vi "S8300E_BP_VLAN_WIH.vi"() -> ()   [LabVIEW 2011]
panel:
  out "PreLog1":string
  out "prelog2":string
  out "log2":string
  out "FinalLog1":string
  out "LOG1":string
  out "Finallog2":string
  out "Test CMD":T1(array[cluster])
  out "Init CMD":T2(array[cluster])
  out "VISA Handle Array":refnum<visa-resource-name>[](array[refnum])
  out "VISA6":refnum<visa-resource-name>
  out "VISA9":refnum<visa-resource-name>
  out "BEGIN TIME":u32
  out "進行狀況":string
  # "Error Code:BP-VLAN"
  # "S8300E BackPlane  VLAN"
  # "2015-5-28"
  # "PC Com9 Baud  115200 -->S8300E MB\nPC COM6 Baud 115200 -->Test Board UART"
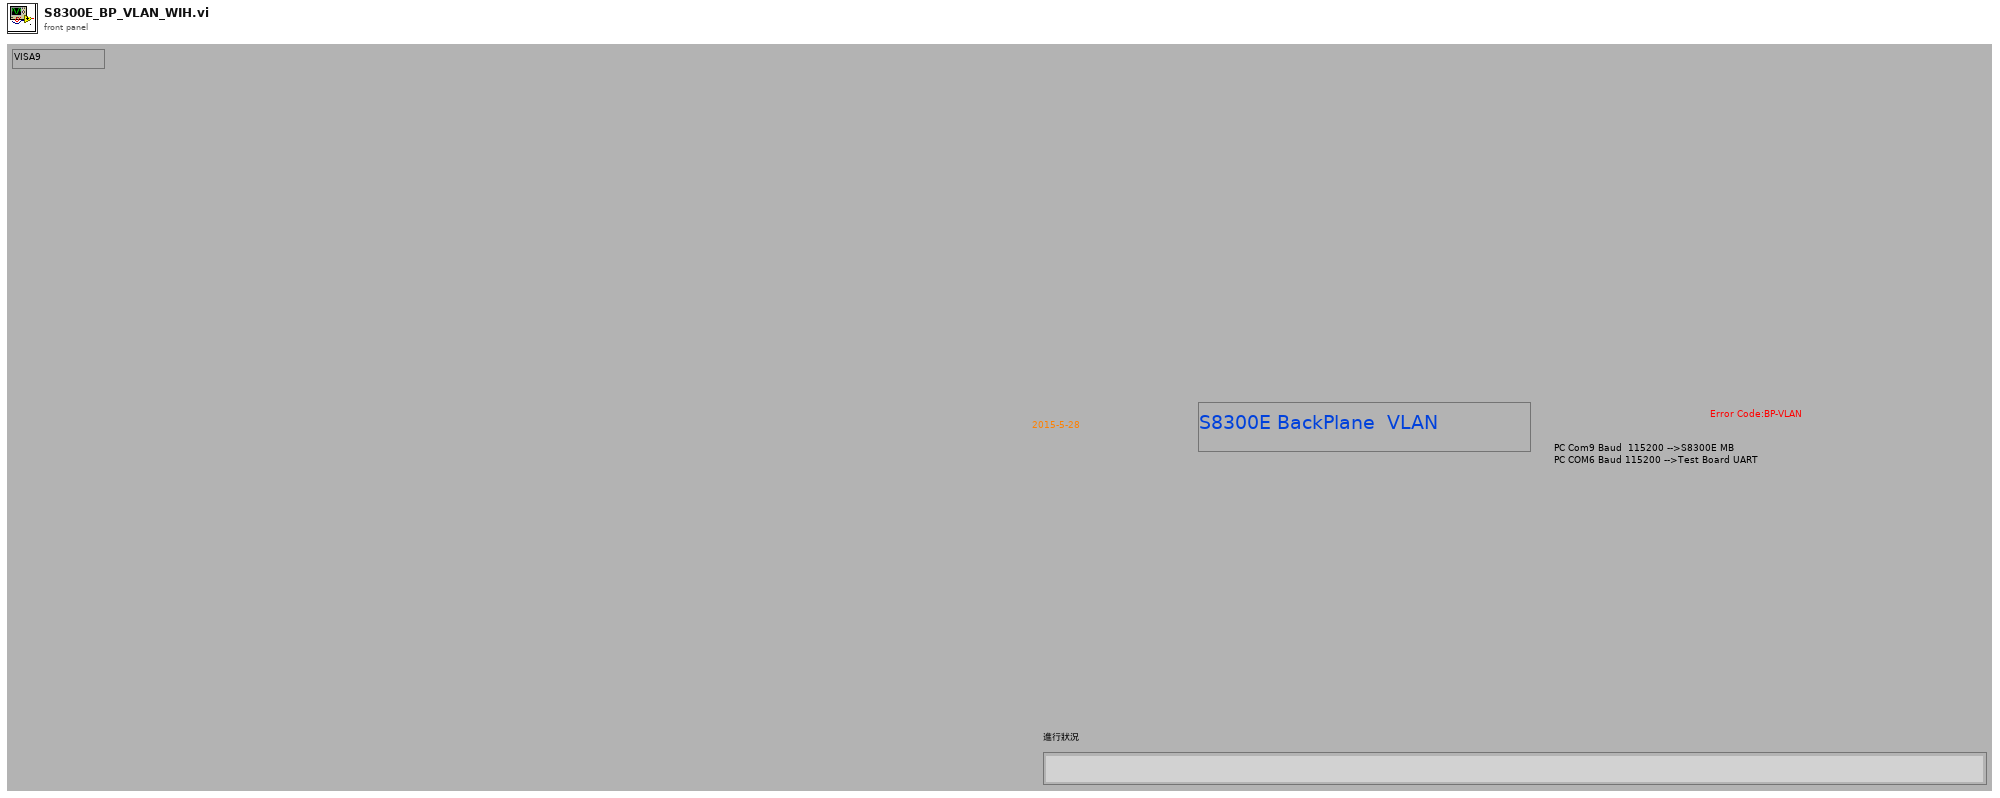
[diagram p1: front panel]
types:
  T1 = cluster{"VISA9":refnum<visa-resource-name>, "Find this String":string, "Find this String":string, "Find this String":string}[]
  T2 = cluster{"Find this String":string, "Find this String":string, "Find this String":string}[]
  T3 = cluster{string, "Find this String":string, "Find this String":string}
  T4 = cluster{"VISA6":refnum<visa-resource-name>, string, "Find this String":string, "Find this String":string}
  T5 = cluster{"VISA9":refnum<visa-resource-name>, string, "Find this String":string, "Find this String":string}
  T6 = cluster{string, "Find this String":string, "Find this String":string}[]
  T7 = cluster{"VISA6":refnum<visa-resource-name>, string, "Find this String":string, "Find this String":string}[]
  T8 = cluster{"Find this String":string, "Find this String":string, "Find this String":string}
  T9 = cluster{"VISA9":refnum<visa-resource-name>, "Find this String":string, "Find this String":string, "Find this String":string}
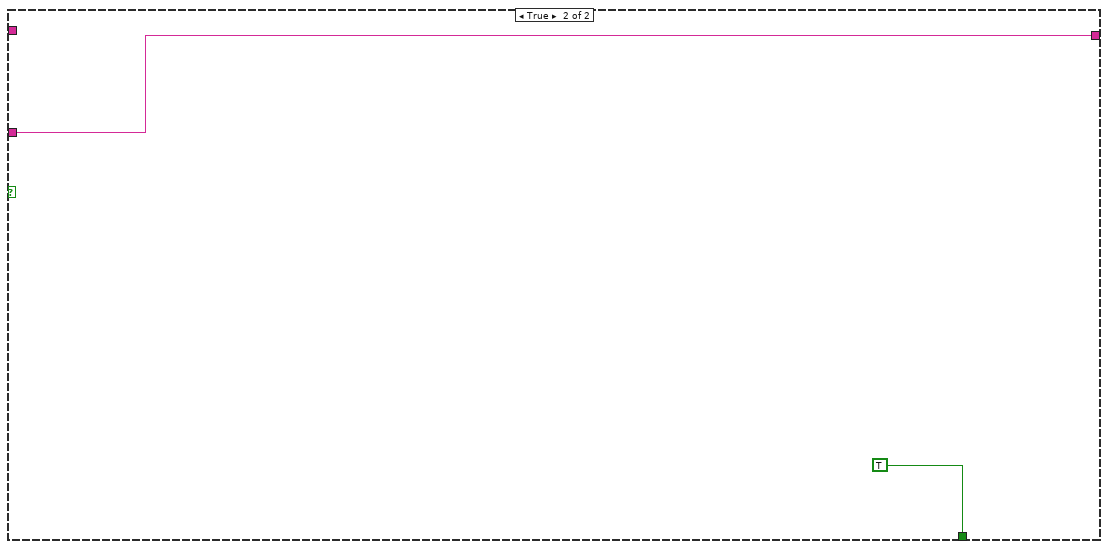
[diagram p4: hidden frame]
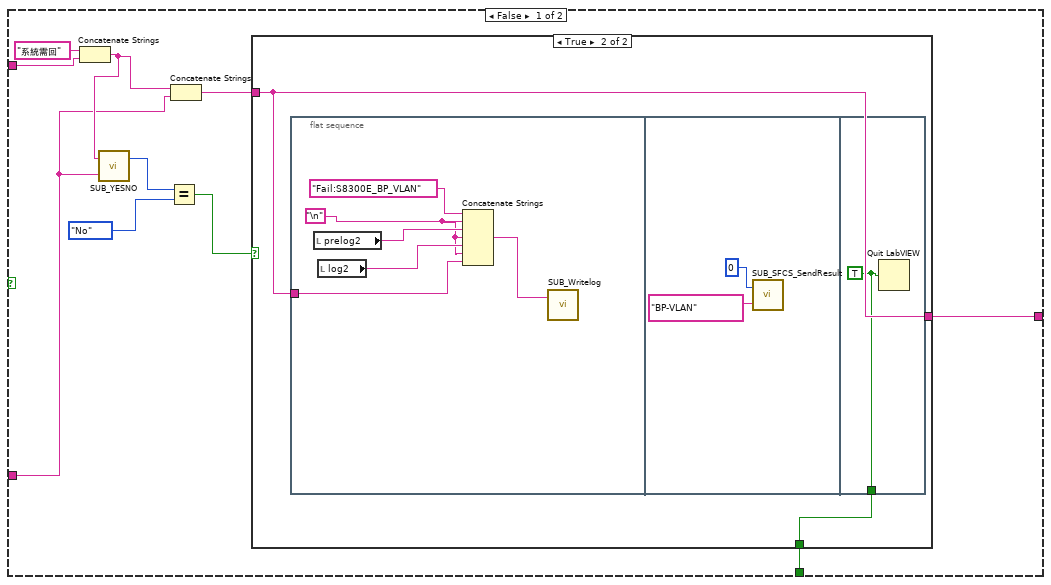
[diagram p5: hidden frame]
diagram:
  n1 = flat-sequence {
    tunnel: [w13] -> w2
    tunnel: w2 -> [w16]
    tunnel: [w183] -> w1
    tunnel: w1 -> [w184]
    frame #0 {
      n2 = Tick Count (ms)() -> (millisecond timer value=→"BEGIN TIME":u32)
    }
    frame #1 {
      n3 = Request Deallocation(TRUE ("flag")) -> ()
      n4 = property on="進行狀況" class="Str"("Blinking"=TRUE) -> ()  [unwired: 2 in, 2 out]
      "進行狀況" <- "進入測試準備中...." ("進行狀況")
    }
    frame #2 {
      n5 = call "SUB_SearchFile_inFolder.vi"("Search Filename in Folder"="S8300E_sfcs_misc.txt") -> ("File Existing True/Flase"=w7:bool)  [unwired: 1 in]
      n6 = case shown="False" w7 {
        frame False {
          n7 = flat-sequence {
            frame #0 {
              n8 = call "Display Message to User"() -> ()  [unwired: 10 in, 2 out]
            }
            frame #1 {
              n9 = call "SUB_Writelog.vi"("Pass/Fail"="Fail:S8300E_BP_VLAN") -> ()  [unwired: 2 in]
            }
            frame #2 {
              n10 = Quit LabVIEW(quit? (T)=TRUE) -> ()
            }
          }
        }
        frame True {
        }
      }
    }
    frame #3 {
      n11 = call "SUB_COM1_CLOSE.vi"("VISA resource name"=refnum<visa-resource-name> "COM6") -> ()  [unwired: 3 in]
    }
    frame #4 {
      n12 = call "SUB_COM1_CLOSE.vi"("VISA resource name"=refnum<visa-resource-name> "COM9") -> ()  [unwired: 3 in]
    }
    frame #5 {
      n13 = call "SUB_COM_INIT.vi"("baud rate (9600)"=u32 115200, "VISA resource name"=refnum<visa-resource-name> "COM6") -> ("VISA resource name out"=w13:refnum<visa-resource-name>)  [unwired: 1 out]
      "VISA6" <- w13
    }
    frame #6 {
      n14 = call "SUB_COM9_INIT.vi"("baud rate"=u32 115200) -> ("VISA resource name out"=w18:refnum<visa-resource-name>)  [unwired: 1 in, 1 out]
      "VISA9" <- w18
      n15 = Build Array(w16, w18) -> (→"VISA Handle Array":refnum<visa-resource-name>[])
    }
    frame #7 {
      n16 = local read "VISA9"() -> (w131:refnum<visa-resource-name>)
      n17 = local read "VISA9"() -> (w119:refnum<visa-resource-name>)
      n18 = local read "VISA9"() -> (w102:refnum<visa-resource-name>)
      n19 = local read "VISA6"() -> (w109:refnum<visa-resource-name>)
      n20 = local read "VISA9"() -> (w41:refnum<visa-resource-name>)
      n21 = Concatenate Strings("DT1" ("Find this String"), "\r") -> (w127:string)
      n22 = local read "VISA6"() -> (w25:refnum<visa-resource-name>)
      n23 = Concatenate Strings("VT0" ("Find this String"), "\r") -> (w33:string)
      n24 = Concatenate Strings("VT1" ("Find this String"), "\r") -> (w38:string)
      n25 = Concatenate Strings("VT0" ("Find this String"), "\r") -> (w124:string)
      n26 = Concatenate Strings("VT1" ("Find this String"), "\r") -> (w128:string)
      n27 = Concatenate Strings("VT1" ("Find this String"), "\r") -> (w113:string)
      n28 = local read "VISA6"() -> (w123:refnum<visa-resource-name>)
      n29 = Concatenate Strings("DT1" ("Find this String"), "\r") -> (w28:string)
      n30 = Concatenate Strings("PT1" ("Find this String"), "\r") -> (w116:string)
      n31 = Concatenate Strings("VT0" ("Find this String"), "\r") -> (w110:string)
      n32 = Concatenate Strings("VT1" ("Find this String"), "\r") -> (w96:string)
      n33 = Concatenate Strings("./bac.sh -a", "\r") -> (w105:string)
      n34 = Concatenate Strings("PT2" ("Find this String"), "\r") -> (w99:string)
      n35 = Concatenate Strings("DT1" ("Find this String"), "\r") -> (w129:string)
      n36 = Concatenate Strings("./bac.sh -v", "\r") -> (w108:string)
      n37 = Concatenate Strings("./bac.sh -a", "\r") -> (w139:string)
      n38 = Concatenate Strings("VT0" ("Find this String"), "\r") -> (w93:string)
      n39 = Concatenate Strings("./bac.sh -v", "\r") -> (w122:string)
      n40 = Concatenate Strings("./bac.sh -v", "\r") -> (w91:string)
      n41 = Concatenate Strings("./bac.sh -a", "\r") -> (w46:string)
      n42 = Bundle(w129, "Find this String"="DT1: Pass", "Find this String"="Checking COM6 Function...") -> (w134:T3)  [unwired: 1 in]
      n43 = Bundle("\r", "Find this String"="s8300e_func_test", "Find this String"="Checking COM9 Function") -> (w133:T3)  [unwired: 1 in]
      n44 = local read "VISA6"() -> (w92:refnum<visa-resource-name>)
      n45 = Bundle("VISA6"=w123, w128, "Find this String"="VT1: Pass", "Find this String"="G450 Output Signal Pattern VT1") -> (w87:T4)  [unwired: 1 in]
      n46 = Bundle("VISA9"=w131, w139, "Find this String"="PASSED", "Find this String"="Set VLAN IP Address Interrupt Acknowledge") -> (w74:T5)  [unwired: 1 in]
      n47 = Bundle("VISA9"=w41, w46, "Find this String"="PASSED", "Find this String"="Set VLAN IP Address Interrupt Acknowledge") -> (w24:T5)  [unwired: 1 in]
      n48 = Bundle("VISA6"=w123, w124, "Find this String"="VT0: Pass", "Find this String"="G450 Output Signal Pattern VT0") -> (w86:T4)  [unwired: 1 in]
      n49 = Bundle("VISA9"=w102, w105, "Find this String"="PASSED", "Find this String"="Set VLAN IP Address Interrupt Acknowledge") -> (w80:T5)  [unwired: 1 in]
      n50 = Bundle("VISA6"=w25, w28, "Find this String"="DT1: Pass", "Find this String"="G450 Output Signal Pattern DT1") -> (w23:T4)  [unwired: 1 in]
      n51 = Bundle("VISA6"=w123, w127, "Find this String"="DT1: Pass", "Find this String"="G450 Output Signal Pattern DT1") -> (w88:T4)  [unwired: 1 in]
      n52 = Bundle("VISA6"=w109, w113, "Find this String"="VT1: Pass", "Find this String"="G450 Output Signal Pattern VT1") -> (w83:T4)  [unwired: 1 in]
      n53 = Bundle("VISA6"=w25, w33, "Find this String"="VT0: Pass", "Find this String"="G450 Output Signal Pattern VT0") -> (w22:T4)  [unwired: 1 in]
      n54 = Bundle("VISA6"=w25, w38, "Find this String"="VT1: Pass", "Find this String"="G450 Output Signal Pattern VT1") -> (w21:T4)  [unwired: 1 in]
      n55 = Bundle("VISA6"=w109, w116, "Find this String"="PT1: Pass", "Find this String"="G450 Output Signal Pattern PT1") -> (w84:T4)  [unwired: 1 in]
      n56 = Bundle("VISA6"=w109, w110, "Find this String"="VT0: Pass", "Find this String"="G450 Output Signal Pattern VT0") -> (w82:T4)  [unwired: 1 in]
      n57 = Bundle("VISA9"=w119, w122, "Find this String"="PASSED=0x00", "Find this String"="Get VLAN address") -> (w85:T5)  [unwired: 1 in]
      n58 = Bundle("VISA6"=w92, w99, "Find this String"="PT2: Pass", "Find this String"="G450 Output Signal Pattern PT2") -> (w79:T4)  [unwired: 1 in]
      n59 = Bundle("VISA6"=w92, w96, "Find this String"="VT1: Pass", "Find this String"="G450 Output Signal Pattern VT1") -> (w78:T4)  [unwired: 1 in]
      n60 = Bundle("VISA9"=w102, w108, "Find this String"="PASSED=0x1a", "Find this String"="Get VLAN address") -> (w81:T5)  [unwired: 1 in]
      n61 = Bundle("VISA6"=w92, w93, "Find this String"="VT0: Pass", "Find this String"="G450 Output Signal Pattern VT0") -> (w77:T4)  [unwired: 1 in]
      n62 = Bundle("VISA9"=w41, w91, "Find this String"="PASSED=0x15", "Find this String"="Get VLAN address") -> (w76:T5)  [unwired: 1 in]
      n63 = Build Array(w134, w133) -> (→"Init CMD":T6)
      n64 = Build Array(w74, w88, w87, w86, w74, w85, w84, w83, w82, w81, w80, w79, w78, w77, w76, w24, w23, w22, w21) -> (→"Test CMD":T7)
    }
    frame #8 {
      n65 = while {
        shift-right: [w155] -> _
        shift-left: "" -> [w156]
        i -> [w160]
        stop <- w161 stop-if-true
        w154 = "Fail" ("Find this String")
        n66 = local read "VISA6"() -> (w149:refnum<visa-resource-name>)
        n67 = Greater Or Equal?(x=w160, y=3) -> (x >= y?=w158:bool)
        n68 = Tick Count (ms)() -> (millisecond timer value=w151:u32)
        n69 = call "SUB_WR_COM1_CbyCFindString_timeout.vi"("Begin time"=w151, "Find this String"=w154, "Timeout Seccond"=3.0, "cmd string"="\r", "duplicate VISA resource name 2"=w149) -> ("Output String"=w157:string, "Found String"=w153:bool)  [unwired: 2 out]
        n70 = Concatenate Strings(w156, w157) -> (w155:string)
        n71 = call "SUB_FindSpecificString.vi"("Find this String"=w154, "String data"=w155) -> ("Found"=w152:bool)  [unwired: 2 in, 1 out]
        n72 = Or(x=w153, y=w152) -> (x .or. y?=w150:bool)
        n73 = Or(x=w150, y=w158) -> (x .or. y?=w161:bool)
      }
    }
    frame #9 {
      n74 = local read "VISA6"() -> (w164:refnum<visa-resource-name>)
      n75 = call "SUB_COM_FLUSH_TXRX.vi"("VISA resource name"=w164) -> ()  [unwired: 2 in, 1 out]
    }
    frame #10 {
      n76 = while {
        shift-right: [w169] -> _
        shift-left: "" -> [w175]
        i -> [w170]
        stop <- w166 stop-if-true
        w168 = "DT1: Pass" ("Find this String")
        n77 = local read "VISA6"() -> (w179:refnum<visa-resource-name>)
        n78 = Concatenate Strings("DT1" ("string"), "\r") -> (w180:string)
        n79 = Greater Or Equal?(x=w170, y=3) -> (x >= y?=w173:bool)
        n80 = Tick Count (ms)() -> (millisecond timer value=w177:u32)
        n81 = call "SUB_WR_COM1_CbyCFindString_timeout.vi"("Begin time"=w177, "Find this String"=w168, "Timeout Seccond"=3.0, "cmd string"=w180, "duplicate VISA resource name 2"=w179) -> ("Output String"=w176:string, "Found String"=w167:bool)  [unwired: 2 out]
        n82 = Concatenate Strings(w175, w176) -> (w169:string)
        n83 = call "SUB_FindSpecificString.vi"("Find this String"=w168, "String data"=w169) -> ("Found"=w172:bool)  [unwired: 2 in, 1 out]
        n84 = Or(x=w167, y=w172) -> (x .or. y?=w171:bool)
        n85 = Or(x=w171, y=w173) -> (x .or. y?=w166:bool)
      }
    }
    frame #11 {
      n86 = Tick Count (ms)() -> (millisecond timer value=w183:u32)
    }
    frame #12 {
      n87 = while {
        shift-right: [w195] -> _
        shift-left: "" -> [w196]
        tunnel: w184 -> [w187]
        stop <- w193 stop-if-true
        n88 = local read "VISA9"() -> (w186:refnum<visa-resource-name>)
        n89 = call "SUB_COM1Wrt.vi"("VISA resource name"=w186, "write buffer"="\r") -> ("duplicate VISA resource name"=w199:refnum<visa-resource-name>)  [unwired: 1 in, 1 out]
        n90 = Tick Count (ms)() -> (millisecond timer value=w191:u32)
        n91 = Subtract(x=w191, y=w187) -> (x-y=w190:u32)
        n92 = Greater Or Equal?(x=w190, y=u32 5000) -> (x >= y?=w188:bool)
        n93 = call "SUB_ContinueCom1Read.vi"("Numeric"=1200, "duplicate VISA resource name 2"=w199) -> ("String"=w197:string)  [unwired: 1 in, 2 out]
        n94 = Concatenate Strings(w196, w197) -> (w195:string)
        n95 = call "SUB_FindSpecificString.vi"("Find this String"="S8300E", "String data"=w195) -> ("Found"=w192:bool)  [unwired: 2 in, 1 out]
        n96 = Or(x=w192, y=w188) -> (x .or. y?=w193:bool)
      }
    }
    frame #13 {
      n97 = local read "Init CMD"() -> (w204:T2)
      n98 = Array Size(array=w204) -> (size(s)=w203:i32)
      n99 = for {
        N: w203 -> [_]
        shift-right: [w207] -> w201
        shift-left: "" -> [w205]
        i -> [w210]
        n100 = local read "VISA Handle Array"() -> (w213:refnum<visa-resource-name>[])
        n101 = local read "Init CMD"() -> (w211:T2)
        n102 = Index Array(array=w213, index=w210) -> (element=w212:refnum<visa-resource-name>)
        n103 = Index Array(array=w211, index=w210) -> (element=w209:T8)
        n104 = while {
          tunnel: w212 -> [w215]
          tunnel: w209 -> [w228]
          shift-right: [w222] -> w206
          shift-left: "" -> [w221]
          stop <- w229 stop-if-true
          n105 = call "SUB_COM_FLUSH_TXRX.vi"("VISA resource name"=w215) -> ("VISA resource name out"=w214:refnum<visa-resource-name>)  [unwired: 2 in]
          n106 = Tick Count (ms)() -> (millisecond timer value=w223:u32)
          n107 = Unbundle(w228) -> ("Find this String"=w219:string, "Find this String"=w225:string, "Find this String"=w227:string)
          n108 = call "SUB_WR_COM1_CbyCFindString_timeout.vi"("Begin time"=w223, "Find this String"=w225, "Timeout Seccond"=5.0, "cmd string"=w219, "duplicate VISA resource name 2"=w214) -> ("Output String"=w216:string, "Found String"=w224:bool)  [unwired: 2 out]
          n109 = local write "進行狀況"(w227) -> ()
          n110 = Concatenate Strings(w219, "\n", w216, w216) -> (w217:string)
          n111 = case shown="False" w224 {
            tunnel: [w237 TRUE] -> w229
            tunnel: w225 -> [w235 _]
            tunnel: w217 -> [w232 w253]
            tunnel: [w231 w253] -> w220
            frame False {
              n112 = Concatenate Strings("UART無正確反應!需有 " ("Status"), w235, "  字串 " ("Status")) -> (w233:string)
              n113 = call "SUB_YESNO.vi"("Debug View"=w232, "Status"=w233) -> ("yes/no"=w240:enum32{"No Selection", "Yes", "No", "None"})  [unwired: 1 in]
              n114 = Equal?(x=w240, y=enum32{"No Selection", "Yes", "No", "None"}."No") -> (x = y?=w238:bool)
              n115 = Concatenate Strings(w233, w232) -> (w230:string)
              n116 = case shown="True" w238 {
                tunnel: [_ w243] -> w237
                tunnel: [w241 w242] -> w231
                tunnel: w230 -> [w241 w242]
                frame False {
                }
                frame True {
                  n117 = flat-sequence {
                    tunnel: w242 -> [w244]
                    tunnel: [w252] -> w243
                    frame #0 {
                      w245 = "\n"
                      n118 = local read "PreLog1"() -> (w247:string)
                      n119 = local read "LOG1"() -> (w246:string)
                      n120 = Concatenate Strings("Fail:S8300E_BP_VLAN" ("Pass/Fail"), w245, w247, w245, w246, w245, w244) -> (w248:string)
                      n121 = call "SUB_Writelog.vi"("Pass/Fail"=w248) -> ()  [unwired: 2 in]
                    }
                    frame #1 {
                      n122 = call "SUB_SFCS_SendResult.vi"("ErrorCode"="UART", "PASS_Fail (1/0)"=i8 0) -> ()  [unwired: 1 out]
                    }
                    frame #2 {
                      w252 = TRUE ("quit? (T)")
                      n123 = Quit LabVIEW(quit? (T)=w252) -> ()
                    }
                  }
                }
              }
            }
            frame True {
            }
          }
          n124 = Concatenate Strings(w221, w220) -> (w222:string)
          "LOG1" <- w222
        }
        n125 = Concatenate Strings(w205, w206) -> (w207:string)
        "PreLog1" <- w207
      }
      "FinalLog1" <- w201
    }
    frame #14 {
      n126 = local read "Test CMD"() -> (w258:T1)
      n127 = Array Size(array=w258) -> (size(s)=w257:i32)
      n128 = for {
        N: w257 -> [_]
        shift-right: [w260] -> w255
        shift-left: "" -> [w259]
        i -> [w263]
        n129 = while {
          tunnel: w263 -> [w280]
          shift-right: [w273] -> w261
          shift-left: "" -> [w272]
          stop <- w277 stop-if-true
          w269 = "\r"
          n130 = local read "Test CMD"() -> (w281:T1)
          n131 = Index Array(array=w281, index=w280) -> (element=w279:T9)
          n132 = Unbundle(w279) -> ("VISA9"=w264:refnum<visa-resource-name>, "Find this String"=w268:string, "Find this String"=w270:string, "Find this String"=w278:string)
          n133 = call "SUB_COM_FLUSH_TXRX.vi"("VISA resource name"=w264) -> ("VISA resource name out"=w265:refnum<visa-resource-name>)  [unwired: 2 in]
          n134 = local write "進行狀況"(w278) -> ()
          n135 = Tick Count (ms)() -> (millisecond timer value=w275:u32)
          n136 = call "SUB_WR_COM1_CbyCFindString_timeout.vi"("Begin time"=w275, "Find this String"=w270, "Timeout Seccond"=5.0, "cmd string"=w268, "duplicate VISA resource name 2"=w265) -> ("Output String"=w267:string, "Found String"=w274:bool)  [unwired: 2 out]
          n137 = Concatenate Strings(w268, w269, w267, w269) -> (w266:string)
          n138 = case shown="True" w274 {
            tunnel: [w287 TRUE] -> w277
            tunnel: [w285 w304] -> w271
            tunnel: w270 -> [w283 _]
            tunnel: w266 -> [w282 w304]
            frame False {
              n139 = Concatenate Strings("系統需回" ("string"), w283) -> (w286:string)
              n140 = call "SUB_YESNO.vi"("Debug View"=w282, "Status"=w286) -> ("yes/no"=w291:enum32{"No Selection", "Yes", "No", "None"})  [unwired: 1 in]
              n141 = Equal?(x=w291, y=enum32{"No Selection", "Yes", "No", "None"}."No") -> (x = y?=w289:bool)
              n142 = Concatenate Strings(w286, w282) -> (w284:string)
              n143 = case shown="True" w289 {
                tunnel: [_ w294] -> w287
                tunnel: [w292 w293] -> w285
                tunnel: w284 -> [w292 w293]
                frame False {
                }
                frame True {
                  n144 = flat-sequence {
                    tunnel: w293 -> [w296]
                    tunnel: [w303] -> w294
                    frame #0 {
                      w297 = "\n"
                      n145 = local read "prelog2"() -> (w299:string)
                      n146 = local read "log2"() -> (w298:string)
                      n147 = Concatenate Strings("Fail:S8300E_BP_VLAN" ("Pass/Fail"), w297, w299, w297, w298, w297, w296) -> (w295:string)
                      n148 = call "SUB_Writelog.vi"("Pass/Fail"=w295) -> ()  [unwired: 2 in]
                    }
                    frame #1 {
                      n149 = call "SUB_SFCS_SendResult.vi"("ErrorCode"="BP-VLAN", "PASS_Fail (1/0)"=i8 0) -> ()  [unwired: 1 out]
                    }
                    frame #2 {
                      w303 = TRUE ("quit? (T)")
                      n150 = Quit LabVIEW(quit? (T)=w303) -> ()
                    }
                  }
                }
              }
            }
            frame True {
            }
          }
          n151 = Concatenate Strings(w272, w271) -> (w273:string)
          "log2" <- w273
        }
        n152 = Concatenate Strings(w259, w261) -> (w260:string)
        "prelog2" <- w260
      }
      "Finallog2" <- w255
    }
    frame #15 {
      n153 = call "SUB_COM1_CLOSE.vi"("VISA resource name"=refnum<visa-resource-name> "COM6") -> ()  [unwired: 3 in]
    }
    frame #16 {
      w309 = "***Not Good ***" ("replace string (\"\")")
      w314 = "\n"
      n154 = local read "Finallog2"() -> (w315:string)
      n155 = local read "FinalLog1"() -> (w316:string)
      n156 = local read "BEGIN TIME"() -> (w320:u32)
      n157 = Tick Count (ms)() -> (millisecond timer value=w319:u32)
      n158 = call "SUB_CAL_TESTTIME.vi"("Test Item name"="S8300E_BP_VLAN", "Stop tick time"=w319, "Start tick time"=w320) -> ("Test Time output"=w313:string)  [unwired: 2 in]
      n159 = call "SUB_COM1_CLOSE.vi"("VISA resource name"=refnum<visa-resource-name> "COM9") -> ()  [unwired: 3 in]
      n160 = Concatenate Strings("Pass:S8300E_BP_VLAN", w314, w316, w314, w315, w314, w313) -> (w308:string)
      n161 = call "SUB_SEARCH_REPLACE_STR.vi"("replace string (\"\")"=w309, "search string"="FAILED", "input string"=w308) -> ("result string"=w311:string)  [unwired: 2 in]
      n162 = call "SUB_SEARCH_REPLACE_STR.vi"("replace string (\"\")"=w309, "search string"="FAIL", "input string"=w311) -> ("result string"=w307:string)  [unwired: 2 in]
      n163 = call "SUB_Writelog.vi"("Pass/Fail"=w307) -> ()  [unwired: 2 in]
    }
    frame #17 {
      n164 = Quit LabVIEW(quit? (T)=TRUE ("stop? (T)")) -> ()
    }
  }
